vi "SimpleMotorFF_Ka_AutoTune.vi"(7 "SimpleMotorFeedforward_KaTune_Pack":T1, 8 "PassThroughTime":dbl=-1.0, 9 "Run Test":bool, 10 "CO Control Output":dbl, 11 "PV ProcessVariable":dbl) -> (0 "Error":bool, 1 "Ka Calc":dbl=-1.0, 2 "Test Complete":bool, 3 "SP Setpoint":dbl=-1.0, 4 "Ka StdDev":dbl=-1.0, 5 "State":i32, 6 "Samples":i32)   [LabVIEW 2019, in "Trajectory_Library.lvlib"]
doc: "This function will ramp the SP up and down while collecting data. Once the ramp is complete Ka will be calculated.\n\nInputs: \n -- PackedParams -- SimpleMotorFF_KA_Tune_Params -- Data cluster containing the parameters defining the test.\n -- PV ProcessVariable -- Double -- The measured variable.\n -- CO Control Output -- Double -- The actuator output demand\n -- Run Test -- Boolean -- When TRUE, run the test.\n -- Pass Through Time -- Double -- Current time (seconds). If not specified, the FPGA time will be read and used.\n\nOutputs:\n -- SP Setpoint -- Double - The desired while performing the test. When not testing the value is set to zero.\n -- Test Complete -- Boolean -- TRUE indicates tht the test has completed and a new Ka value has been calculationed.\n -- Ka Calc -- Double -- Newly calculated Ka value. Only valid when Test Complete is TRUE. This value is averaged from a number of individual Ka calculations made between the Min and Max eval SP values.\n -- Error -- Boolean -- TRUE indicates an error has occured.\n -- Ka Std Dev -- Double -- Standard deviation of the array of Ka used to calculate the average Ka.\n -- Samples -- Double -- The number of samples used to calculte Ka."
uses:
  Trajectory_Library.lvlib
  TypeDef/SIMPLE_MOTOR_FF_KA_TUNE_PARAMS.ctl
  TimeInterpDouble_CleanUp.vi
  MathUtil_Interpolate.vi
  MathUtil_Clamp.vi
  <vilib>/gmath/interp.llb/Search Ordered Table.vi
  <vilib>/Analysis/NI_AALBase.lvlib
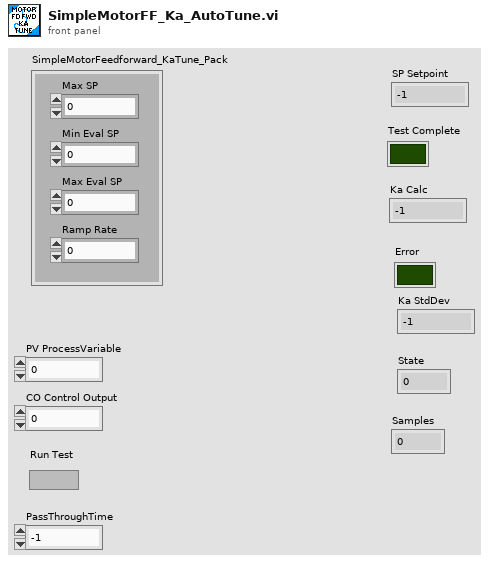
[diagram p1: front panel]
types:
  T1 = typedef "Trajectory_Library.lvlib/SIMPLE_MOTOR_FF_KA_TUNE_PARAMS.ctl" = cluster{"Max SP":dbl, "Min Eval SP":dbl, "Max Eval SP":dbl, "Ramp Rate":dbl}
  T2 = typedef "Trajectory_Library.lvlib/TIME_INTERPOLATABLE_DOUBLE.ctl" = cluster{"TimeStamps":dbl[], "DoubleValue":dbl[], "Min_TimeStamp":dbl, "Max_TimeStamp":dbl, "ItemCount":i32, "MaxBufferTime":dbl}
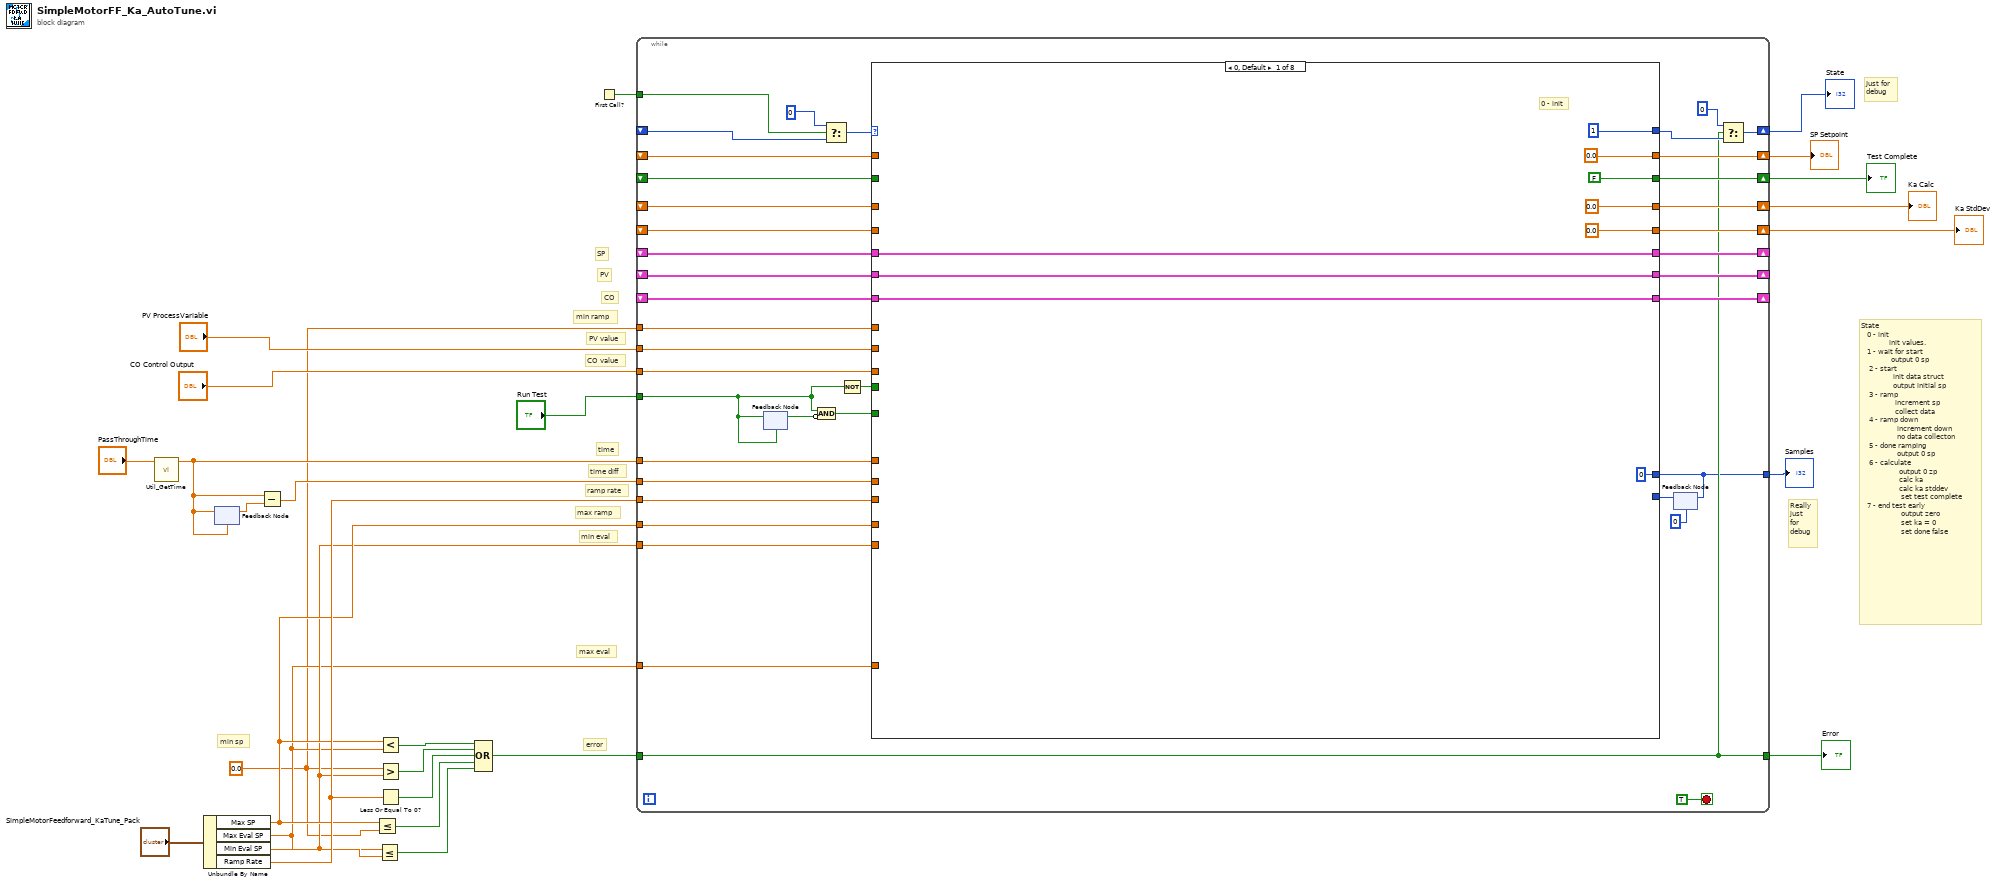
[diagram p0: block diagram]
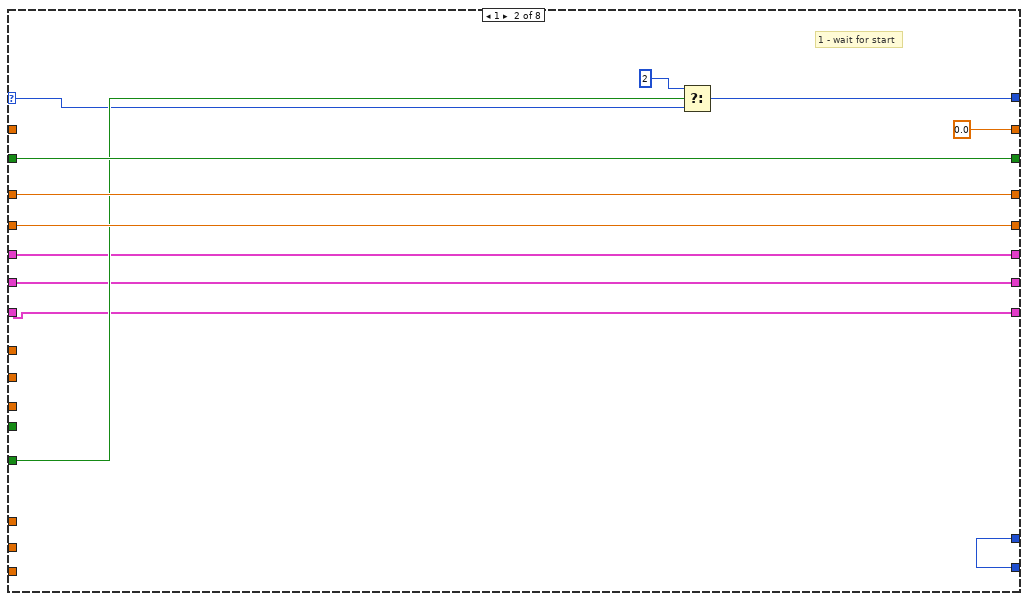
[diagram p2: hidden frame]
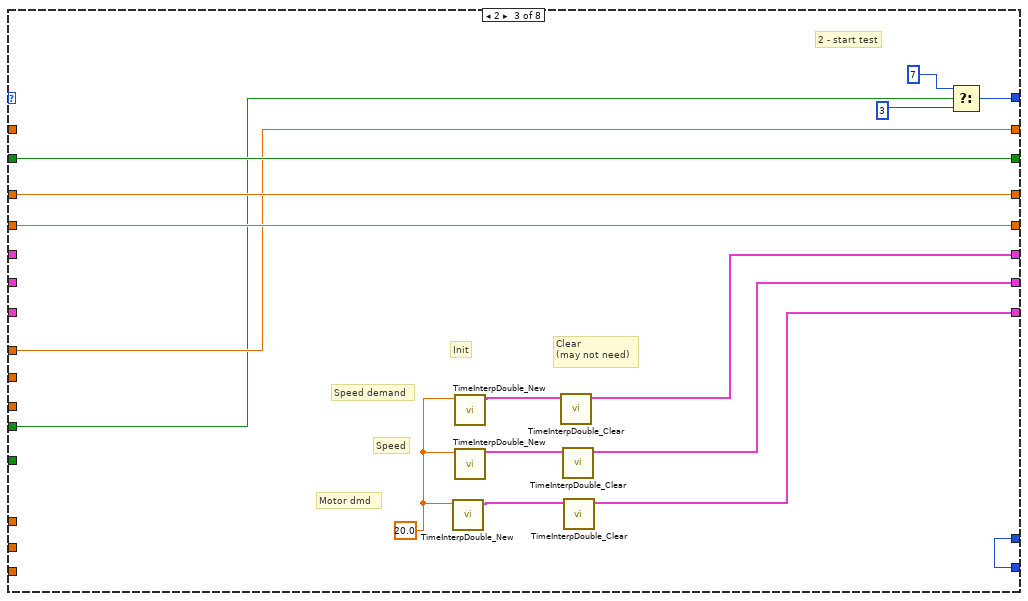
[diagram p3: hidden frame]
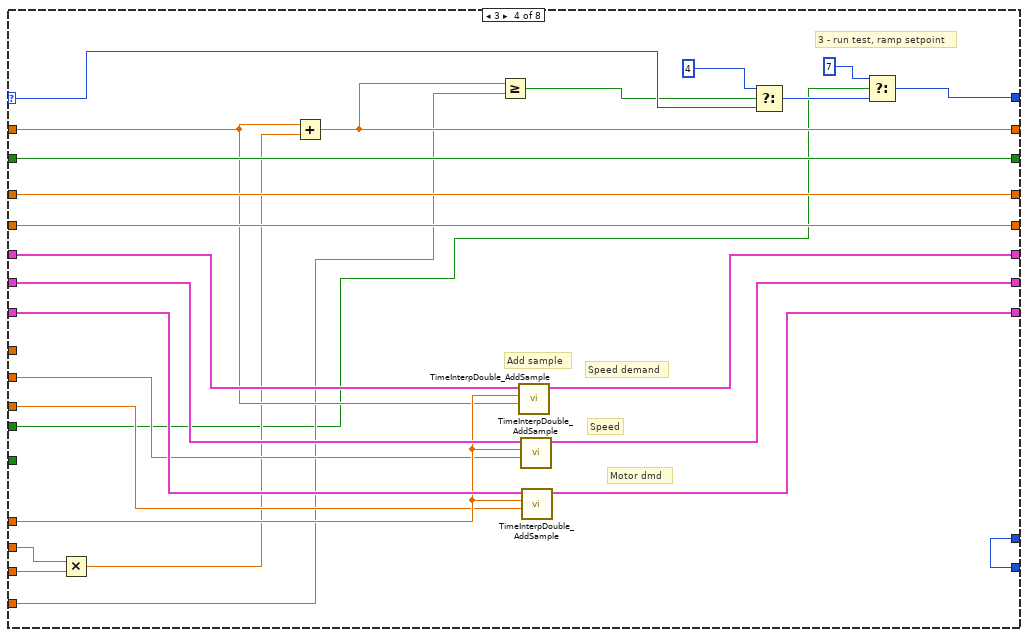
[diagram p4: hidden frame]
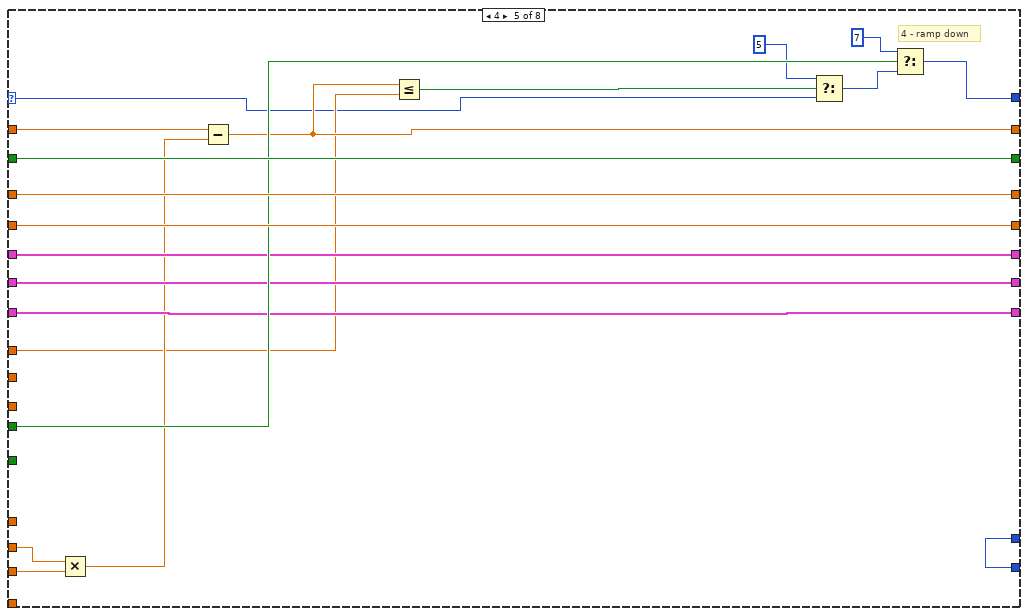
[diagram p5: hidden frame]
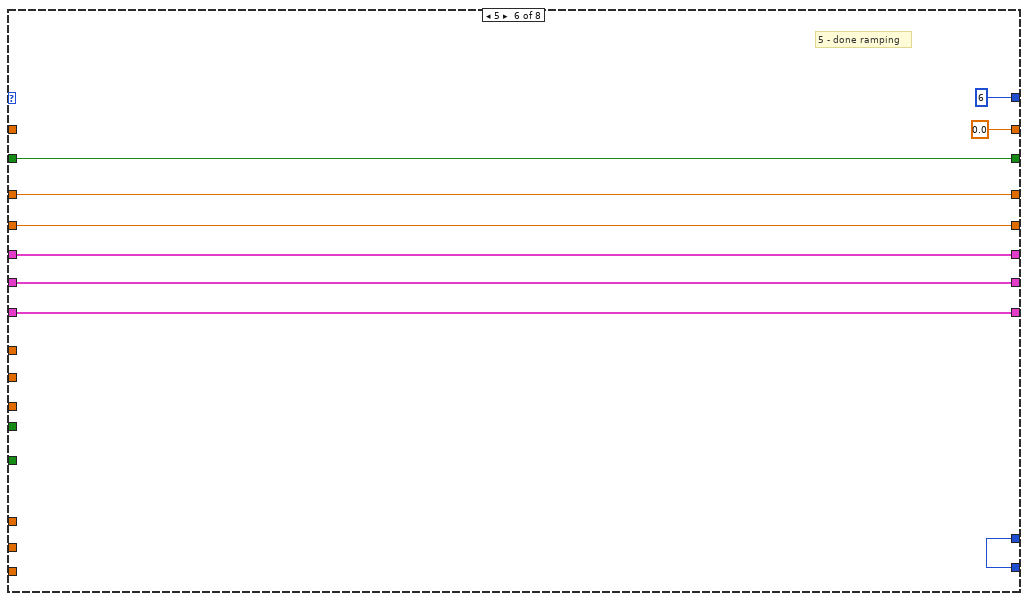
[diagram p6: hidden frame]
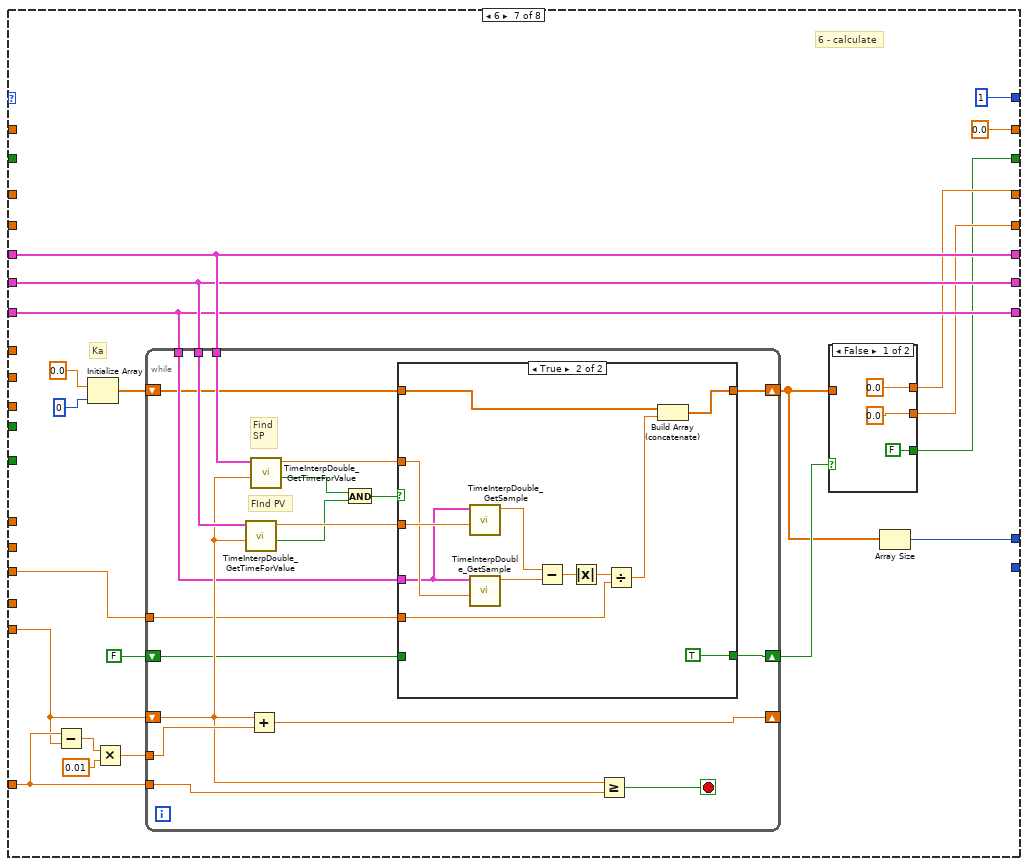
[diagram p7: hidden frame]
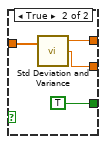
[diagram p8: hidden frame]
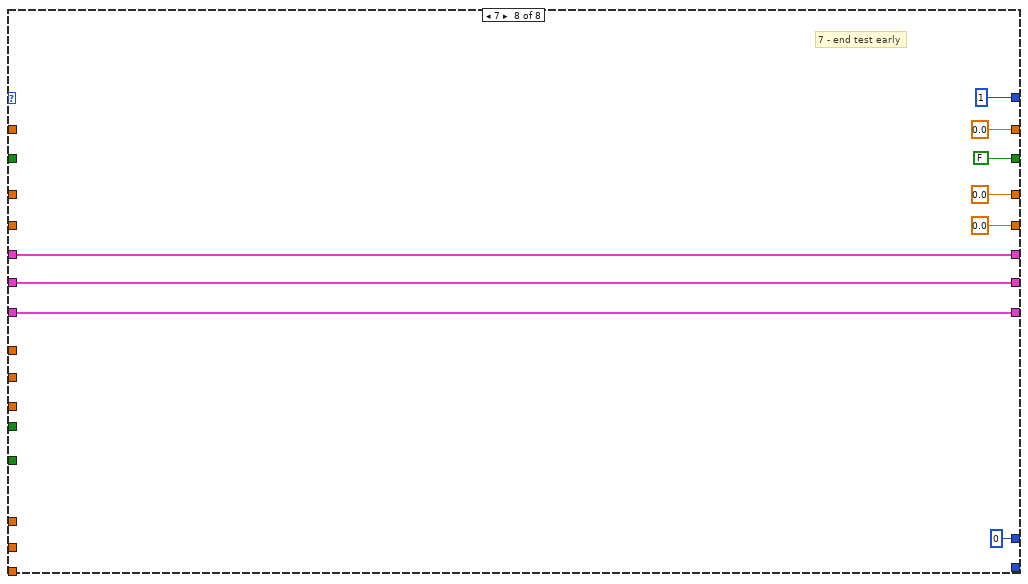
[diagram p10: hidden frame]
diagram:
  w3 = 0.0
  # "Just for\ndebug"
  # "Really\njust\nfor \ndebug"
  # "error"
  # "min eval"
  # "max eval"
  # "max ramp"
  # "min ramp"
  # "CO value"
  # "PV value"
  # "min sp"
  # "time diff"
  # "time"
  # "ramp rate"
  # "CO"
  # "PV"
  # "SP"
  # "State\n   0 - init\n              init values.\n   1 - wait for start\n               output 0 sp\n    2 - start\n                init data struct\n                output initial sp\n    3 - ramp\n                 increment sp\n                 collect data\n    4 - ramp down\n                  increment down\n                  no data collecton\n    5 - done ramping \n                  output 0 sp\n    6 - calculate\n                   output 0 zp\n                   calc ka\n                   calc ka stddev\n                    set test complete \n   7 - end test early\n                    output zero\n                    set ka = 0\n                    set done false"
  n1 = call "Util_GetTime.vi"("Pass_Through_Time"="PassThroughTime") -> ("FPGA_Time_Seconds"=w9:dbl)  [unwired: 8 in, 2 out]
  n2 = Unbundle By Name("SimpleMotorFeedforward_KaTune_Pack") -> ("Max SP"=w6:dbl, "Max Eval SP"=w4:dbl, "Min Eval SP"=w5:dbl, "Ramp Rate"=w11:dbl)
  n3 = feedback-in #1(w9) -> ()
  n4 = feedback #1(w9) -> (w12:dbl)
  n5 = Subtract(x=w9, y=w12) -> (x-y=w10:dbl)
  n6 = Less Or Equal?(x=w6, y=w3) -> (x <= y?=w23:bool)
  n7 = Less Or Equal?(x=w4, y=w5) -> (x <= y?=w22:bool)
  n8 = Less?(x=w6, y=w4) -> (x < y?=w26:bool)
  n9 = Greater?(x=w3, y=w5) -> (0:w25:bool)
  n10 = Less Or Equal To 0?(x=w11) -> (x <= 0?=w24:bool)
  n11 = Compound Arithmetic op=OR(w26, w25, w24, w23, w22) -> (w16:bool)
  n12 = First Call?() -> (First Call?: T/F=w15:bool)
  n13 = while {
    shift-right: [w65] -> w17
    shift-left: _ -> [w48]
    shift-right: [w64] -> w18
    shift-left: _ -> [w61]
    shift-right: [w63] -> w19
    shift-left: _ -> [w60]
    shift-right: [w62] -> w21
    shift-left: _ -> [w59]
    tunnel: w15 -> [w56]
    tunnel: "Run Test" -> [w36]
    shift-right: [w34] -> w2
    shift-left: _ -> [w55]
    shift-right: [w54] -> _
    shift-left: _ -> [w51]
    shift-right: [w53] -> _
    shift-left: _ -> [w50]
    shift-right: [w52] -> _
    shift-left: _ -> [w49]
    tunnel: w3 -> [w47]
    tunnel: w11 -> [w46]
    tunnel: w10 -> [w45]
    tunnel: w9 -> [w44]
    tunnel: "PV ProcessVariable" -> [w43]
    tunnel: "CO Control Output" -> [w42]
    tunnel: w6 -> [w41]
    tunnel: w5 -> [w40]
    tunnel: w4 -> [w39]
    tunnel: w16 -> [w31]
    tunnel: [w31] -> w20
    tunnel: [w30] -> w1
    stop <- TRUE stop-if-true
    n14 = feedback-in #2(w36) -> ()
    n15 = feedback #2(w36) -> (w66:bool)
    n16 = Compound Arithmetic op=AND(w36, invert w66) -> (w37:bool)
    n17 = Select(t=0, s=w56, f=w55) -> (s? t:f=w58:i32)
    n18 = Not(x=w36) -> (.not. x?=w35:bool)
    n19 = feedback #3(0) -> (w28:i32)
    n20 = case shown="0, Default" w58 {
      selector: w58 -> [_ w82 _ w112 w131 _ _ _]
      tunnel: w37 -> [_ w83 _ _ _ _ _ _]
      tunnel: [0.0 ("SetPoint") 0.0 ("SetPoint") w93 w110 w134 0.0 ("Min SP") 0.0 ("Min SP") 0.0 ("Min SP")] -> w65
      tunnel: [FALSE ("Test Complete") w86 w103 w129 w149 w158 w161 FALSE ("Test Complete")] -> w64
      tunnel: [0.0 ("Ka Calc") w85 w102 w128 w148 w157 w165 0.0 ("mean")] -> w63
      tunnel: [0.0 ("Ka StdDev") w84 w101 w127 w147 w156 w164 0.0 ("standard deviation")] -> w62
      tunnel: w61 -> [_ w86 w103 w129 w149 w158 _ _]
      tunnel: w60 -> [_ w85 w102 w128 w148 w157 _ _]
      tunnel: w59 -> [_ w84 w101 w127 w147 w156 _ _]
      tunnel: [1 w80 w92 w106 w145 6 1 1] -> w33
      tunnel: [w70 w79 w96 w124 w143 w153 w169 w225] -> w54
      tunnel: [w69 w78 w95 w123 w142 w152 w168 w224] -> w53
      tunnel: [w68 w77 w94 w122 w141 w151 w167 w223] -> w52
      tunnel: w51 -> [w70 w79 _ w121 w143 w153 w169 w225]
      tunnel: w50 -> [w69 w78 _ w120 w142 w152 w168 w224]
      tunnel: w49 -> [w68 w77 _ w119 w141 w151 w167 w223]
      tunnel: w48 -> [_ _ _ w115 w140 _ _ _]
      tunnel: w47 -> [_ _ w93 _ w133 _ _ _]
      tunnel: w46 -> [_ _ _ w126 w138 _ w166 _]
      tunnel: w45 -> [_ _ _ w125 w139 _ _ _]
      tunnel: w44 -> [_ _ _ w118 _ _ _ _]
      tunnel: w43 -> [_ _ _ w117 _ _ _ _]
      tunnel: w42 -> [_ _ _ w116 _ _ _ _]
      tunnel: w41 -> [_ _ _ w109 _ _ _ _]
      tunnel: w40 -> [_ _ _ _ _ _ w176 _]
      tunnel: w39 -> [_ _ _ _ _ _ w177 _]
      tunnel: w35 -> [_ _ w89 w105 w144 _ _ _]
      tunnel: [0 w76 w88 w104 w130 w150 w159 0] -> w30
      tunnel: w28 -> [_ w76 w88 w104 w130 w150 _ _]
      frame 0, Default {
        # "0 - init"
      }
      frame 1 {
        # "1 - wait for start"
        n21 = Select(t=2, s=w83, f=w82) -> (s? t:f=w80:i32)
      }
      frame 2 {
        w100 = 20.0 ("MaxTime")
        # "Clear\n(may not need)"
        # "Init"
        # "Motor dmd"
        # "Speed"
        # "Speed demand"
        # "2 - start test"
        n22 = call "TimeInterpDouble_New.vi"("MaxTime"=w100) -> ("TimeInterpDouble"=w97:T2)  [unwired: 10 in]
        n23 = call "TimeInterpDouble_New.vi"("MaxTime"=w100) -> ("TimeInterpDouble"=w99:T2)  [unwired: 10 in]
        n24 = call "TimeInterpDouble_New.vi"("MaxTime"=w100) -> ("TimeInterpDouble"=w98:T2)  [unwired: 10 in]
        n25 = call "TimeInterpDouble_Clear.vi"("in TimeInterpDouble"=w99) -> ("out TimeInterpDouble"=w96:T2)  [unwired: 10 in]
        n26 = call "TimeInterpDouble_Clear.vi"("in TimeInterpDouble"=w98) -> ("out TimeInterpDouble"=w95:T2)  [unwired: 10 in]
        n27 = call "TimeInterpDouble_Clear.vi"("in TimeInterpDouble"=w97) -> ("out TimeInterpDouble"=w94:T2)  [unwired: 10 in]
        n28 = Select(t=7, s=w89, f=3) -> (s? t:f=w92:i32)
      }
      frame 3 {
        # "Add sample"
        # "Motor dmd"
        # "Speed"
        # "Speed demand"
        # "3 - run test, ramp setpoint"
        n29 = Multiply(x=w125, y=w126) -> (x*y=w114:dbl)
        n30 = Add(x=w115, y=w114) -> (x+y=w110:dbl)
        n31 = Greater Or Equal?(x=w110, y=w109) -> (x >= y?=w111:bool)
        n32 = call "TimeInterpDouble_AddSample.vi"("Value"=w115, "TimeStamp"=w118, "in TimeInterpDouble"=w121) -> ("out TimeInterpDouble"=w124:T2)  [unwired: 7 in, 1 out]
        n33 = call "TimeInterpDouble_AddSample.vi"("Value"=w117, "TimeStamp"=w118, "in TimeInterpDouble"=w120) -> ("out TimeInterpDouble"=w123:T2)  [unwired: 7 in, 1 out]
        n34 = call "TimeInterpDouble_AddSample.vi"("Value"=w116, "TimeStamp"=w118, "in TimeInterpDouble"=w119) -> ("out TimeInterpDouble"=w122:T2)  [unwired: 7 in, 1 out]
        n35 = Select(t=4, s=w111, f=w112) -> (s? t:f=w107:i32)
        n36 = Select(t=7, s=w105, f=w107) -> (s? t:f=w106:i32)
      }
      frame 4 {
        # "4 - ramp down"
        n37 = Multiply(x=w139, y=w138) -> (x*y=w137:dbl)
        n38 = Subtract(x=w140, y=w137) -> (x-y=w134:dbl)
        n39 = Less Or Equal?(x=w134, y=w133) -> (x <= y?=w132:bool)
        n40 = Select(t=5, s=w132, f=w131) -> (s? t:f=w135:i32)
        n41 = Select(t=7, s=w144, f=w135) -> (s? t:f=w145:i32)
      }
      frame 5 {
        # "5 - done ramping"
      }
      frame 6 {
        # "Ka"
        # "6 - calculate"
        n42 = Subtract(x=w177, y=w176) -> (x-y=w175:dbl)
        n43 = Initialize Array(0.0 ("element"), 0 ("dimension size")) -> (w172:dbl[])
        n44 = Multiply(x=w175, y=0.01) -> (x*y=w173:dbl)
        n45 = while {
          shift-right: [w201] -> _
          shift-left: w176 -> [w196]
          tunnel: w177 -> [w203]
          tunnel: w173 -> [w202]
          shift-right: [w189] -> w160
          shift-left: w172 -> [w190]
          tunnel: w169 -> [w198]
          tunnel: w168 -> [w197]
          tunnel: w167 -> [w195]
          tunnel: w166 -> [w194]
          shift-right: [w187] -> w162
          shift-left: FALSE -> [w188]
          stop <- w204 stop-if-true
          # "FInd PV"
          # "Find\nSP"
          n46 = call "TimeInterpDouble_GetTimeForValue.vi"("ValueToFind"=w196, "TimeInterpDouble"=w197) -> ("ValueFound"=w192:bool, "TimeStamp"=w200:dbl)  [unwired: 8 in]
          n47 = Add(x=w196, y=w202) -> (x+y=w201:dbl)
          n48 = call "TimeInterpDouble_GetTimeForValue.vi"("ValueToFind"=w196, "TimeInterpDouble"=w198) -> ("ValueFound"=w193:bool, "TimeStamp"=w199:dbl)  [unwired: 8 in]
          n49 = And(x=w193, y=w192) -> (x .and. y?=w191:bool)
          n50 = case shown="True" w191 {
            tunnel: w200 -> [_ w218]
            tunnel: w199 -> [_ w213]
            tunnel: w195 -> [_ w211]
            tunnel: w194 -> [_ w212]
            tunnel: [w206 w208] -> w189
            tunnel: w190 -> [w206 w210]
            tunnel: w188 -> [w205 _]
            tunnel: [w205 TRUE] -> w187
            frame False {
            }
            frame True {
              n51 = call "TimeInterpDouble_GetSample.vi"("TimeStamp"=w218, "TimeInterpDouble"=w211) -> ("OutputDouble"=w214:dbl)  [unwired: 8 in, 1 out]
              n52 = call "TimeInterpDouble_GetSample.vi"("TimeStamp"=w213, "TimeInterpDouble"=w211) -> ("OutputDouble"=w215:dbl)  [unwired: 8 in, 1 out]
              n53 = Subtract(x=w214, y=w215) -> (x-y=w216:dbl)
              n54 = Absolute Value(x=w216) -> (abs(x)=w217:dbl)
              n55 = Divide(x=w217, y=w212) -> (x/y=w209:dbl)
              n56 = Build Array (concatenate)(w210, w209) -> (w208:dbl[])
            }
          }
          n57 = Greater Or Equal?(x=w196, y=w203) -> (x >= y?=w204:bool)
        }
        n58 = case shown="False" w162 {
          tunnel: w160 -> [_ w186]
          tunnel: [0.0 w185] -> w165
          tunnel: [0.0 w184] -> w164
          tunnel: [FALSE TRUE] -> w161
          frame False {
          }
          frame True {
            n59 = call <vilib>:"Std Deviation and Variance.vi"("X"=w186) -> ("mean"=w185:dbl, "standard deviation"=w184:dbl)  [unwired: 1 in, 1 out]
          }
        }
        n60 = Array Size(array=w160) -> (size(s)=w159:i32)
      }
      frame 7 {
        # "7 - end test early"
      }
    }
    n61 = feedback-in #3(w30) -> ()
    n62 = Select(t=0, s=w31, f=w33) -> (s? t:f=w34:i32)
  }
  "SP Setpoint" <- w17
  "Ka Calc" <- w19
  "Ka StdDev" <- w21
  "Error" <- w20
  "Test Complete" <- w18
  "State" <- w2
  "Samples" <- w1
